vi "Close.vi"(8 "error in":errorcluster, 11 "Flow Limit in":refnum<class "Flow Limit.lvclass">) -> (0 "error out":errorcluster, 3 "Flow Limit out":refnum<class "Flow Limit.lvclass">)   [LabVIEW 2023, in "Flow Limit.lvclass"]
uses:
  Flow Limit.lvclass
  Parents/Limit/Limit.lvclass
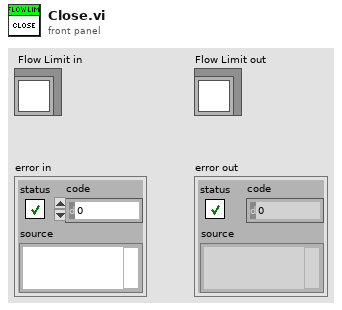
[diagram p1: front panel]
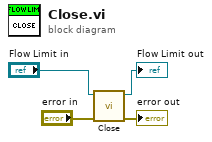
[diagram p0: block diagram]
diagram:
  n1 = call-parent "Close.vi"("error in"="error in", "Limit in"="Flow Limit in") -> ("error out"=→"error out":errorcluster, "Limit out"=→"Flow Limit out":refnum<class "Flow Limit.lvclass">)  [unwired: 8 in]
